vi "VIRCAdll.vi"(8 "error in (no error)":errorcluster, 10 "z":dbl[](array[numeric]), 11 "t":dbl) -> (0 "error out":errorcluster, 3 "ca":dbl)   [LabVIEW 2016]
doc: "subroutine VIRCA (t,z,ca)\n\nCompute third acoustic virial coefficient as a function of temperature\nand composition.\n\nINPUTS:\n t--temperature [K]\n z--composition [array of mol frac]\n\nOUTPUTS:\n ca--third acoustic virial coefficient [(L/mol)^2]"
uses:
  REFPROP.DLL
panel:
  # "REFPROP-VIRCAdll.vi"
  # "void  VIRCAdll(double *t, double *z, double *ca);"
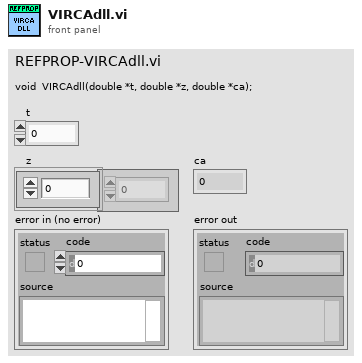
[diagram p1: front panel]
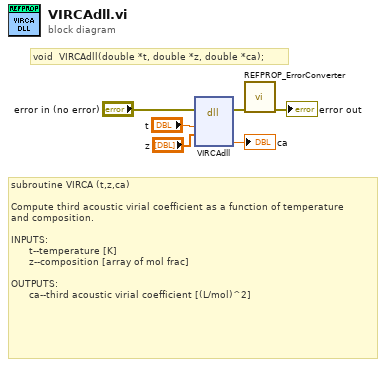
[diagram p0: block diagram]
diagram:
  # "void  VIRCAdll(double *t, double *z, double *ca);"
  # "subroutine VIRCA (t,z,ca)\n\nCompute third acoustic virial coefficient as a function of temperature\nand composition.\n\nINPUTS:\n      t--temperature [K]\n      z--composition [array of mol frac]\n\nOUTPUTS:\n      ca--third acoustic virial coefficient [(L/mol)^2]"
  n1 = dll-call lib="S:/009 - Testing/02 - Performance Testing/REFPROP/REFPROP.*" fn="VIRCAdll"(error in="error in (no error)", "t"="t", "z"="z") -> (error out=w3:errorcluster, "ca"=→"ca":dbl)  [unwired: 6 in, 1 out]
  n2 = call "REFPROP_ErrorConverter.vi"("error in (no error)"=w3) -> ("error out"=→"error out":errorcluster)  [unwired: 10 in]
